vi "FlipFlopJK_1.vi"(9 "K":bool, 10 "Boolean in":bool, 11 "J":bool) -> (2 "Q*":bool, 3 "Boolean out":bool)   [LabVIEW 2018]
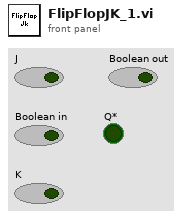
[diagram p1: front panel]
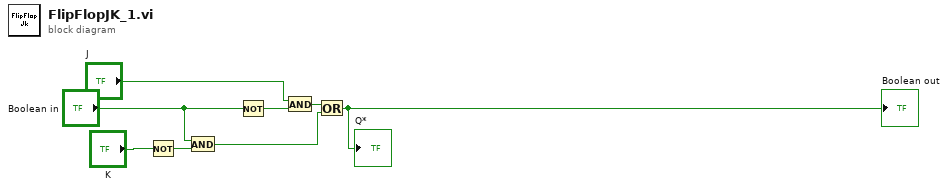
[diagram p0: block diagram]
diagram:
  n1 = Not(x="K") -> (.not. x?=w7:bool)
  n2 = And(x="Boolean in", y=w7) -> (x .and. y?=w2:bool)
  n3 = Not(x="Boolean in") -> (.not. x?=w5:bool)
  n4 = And(x="J", y=w5) -> (x .and. y?=w1:bool)
  n5 = Or(x=w1, y=w2) -> (x .or. y?=→"Q*" →"Boolean out":bool)
